vi "DriveReadEncoder.vi"(8 "error in":errorcluster, 11 "ModualNamePrefix":i32) -> (0 "error out":errorcluster, 2 "SWERVE_DRIVE_MODULE_POSITION":T1={"Distance"=0.0, "Angle"={"VALUE"=0.0, "COS"=1.0, "SIN"=0.0}, "P"=FALSE} {"Angle"."SIN" format="%13.4f"; "Angle"."COS" format="%13.4f"; "Angle"."VALUE" format="%13.4f"}, 3 "SWERVE_DRIVE_MODULE_STATE":T3={"Speed"=0.0, "Angle"={"VALUE"=0.0, "COS"=1.0, "SIN"=0.0}} {"Angle"."SIN" format="%13.4f"; "Angle"."COS" format="%13.4f"; "Angle"."VALUE" format="%13.4f"})   [LabVIEW 2023]
uses:
  <vilib>/Rock Robotics/WPI/ThirdParty/JAS_Junk/TrajLib/TypeDef/SWERVE_DRIVE_MODULE_STATE.ctl
  <vilib>/Rock Robotics/WPI/ThirdParty/JAS_Junk/TrajLib/TypeDef/ROTATION2D.ctl
  <vilib>/Rock Robotics/WPI/ThirdParty/JAS_Junk/TrajLib/TypeDef/SWERVE_DRIVE_MODULE_POSITION.ctl
  <vilib>/Rock Robotics/WPI/ThirdParty/JAS_Junk/TrajLib/Conv_Deg_Radians.vi
  <vilib>/Rock Robotics/WPI/ThirdParty/JAS_Junk/TrajLib/Rotation2d_CreateAngle.vi
  DriveGlobal.vi
  <vilib>/Rock Robotics/WPI/ThirdParty/Phoenix-LabVIEW/CANCoder/CTRE_Phoenix_CANcoder_RefNumRegistryGet.vi
  <vilib>/Rock Robotics/WPI/MotorControl/WPI_MotorControlRefNum Registry Get.vi
  <vilib>/Rock Robotics/WPI/ThirdParty/JAS_Junk/TrajLib/Trajectory_Library.lvlib
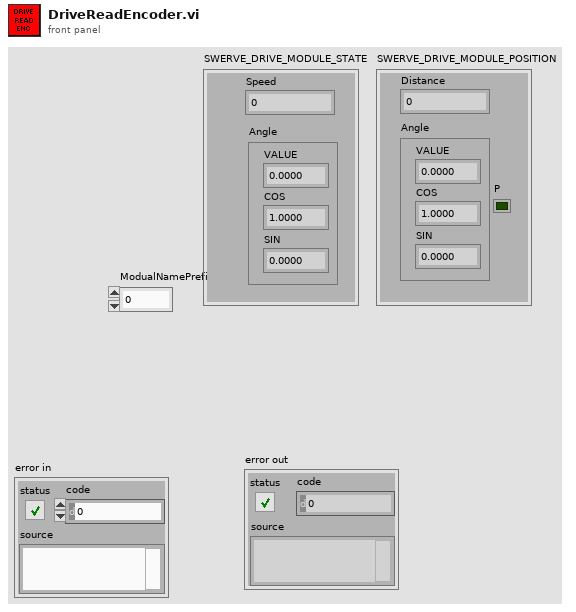
[diagram p1: front panel]
types:
  T1 = typedef "Trajectory_Library.lvlib/SWERVE_DRIVE_MODULE_POSITION.ctl" = cluster{"Distance":dbl, "Angle":T2, "P":bool}
  T2 = typedef "Trajectory_Library.lvlib/ROTATION2D.ctl" = cluster{"VALUE":dbl, "COS":dbl, "SIN":dbl}
  T3 = typedef "Trajectory_Library.lvlib/SWERVE_DRIVE_MODULE_STATE.ctl" = cluster{"Speed":dbl, "Angle":T2}
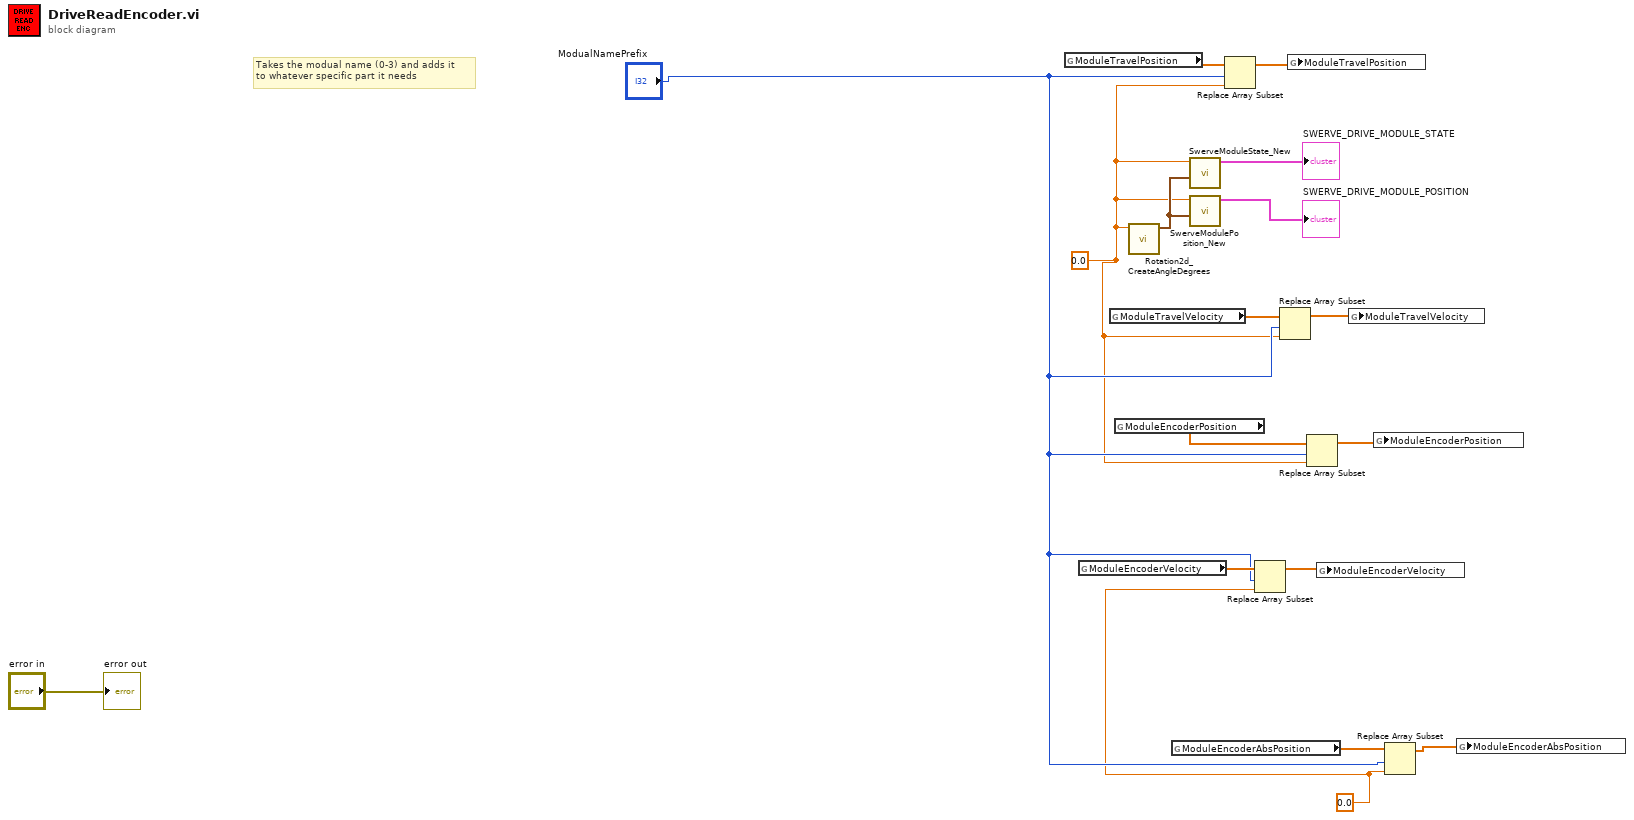
[diagram p0: block diagram]
diagram:
  w2 = 0.0 ("new element/subarray")
  w1 = 0.0 ("new element/subarray")
  # "Takes the modual name (0-3) and adds it \nto whatever specific part it needs"
  n1 = global read "DriveGlobal.vi" "ModuleTravelPosition"() -> (w13:dbl[])
  n2 = global read "DriveGlobal.vi" "ModuleEncoderVelocity"() -> (w7:dbl[])
  n3 = global read "DriveGlobal.vi" "ModuleTravelVelocity"() -> (w11:dbl[])
  n4 = global read "DriveGlobal.vi" "ModuleEncoderPosition"() -> (w9:dbl[])
  n5 = call <vilib>:"Rotation2d_CreateAngleDegrees.vi"("Angle_Degrees"=w2) -> ("ROTATION"=w16:T2)  [unwired: 10 in]
  n6 = global read "DriveGlobal.vi" "ModuleEncoderAbsPosition"() -> (w5:dbl[])
  n7 = call <vilib>:"SwerveModuleState_New.vi"("ROTATION"=w16, "Speed"=w2) -> ("SWERVE_DRIVE_MODULE_STATE"=→"SWERVE_DRIVE_MODULE_STATE":T3)  [unwired: 9 in]
  n8 = call <vilib>:"SwerveModulePosition_New.vi"("ROTATION"=w16, "Distance"=w2) -> ("SWERVE_DRIVE_MODULE_POSITION"=→"SWERVE_DRIVE_MODULE_POSITION":T1)  [unwired: 9 in]
  n9 = Replace Array Subset(array=w13, new element=w2, index="ModualNamePrefix") -> (w12:dbl[])
  n10 = Replace Array Subset(array=w7, new element=w1, index="ModualNamePrefix") -> (w6:dbl[])
  n11 = Replace Array Subset(array=w11, new element=w2, index="ModualNamePrefix") -> (w10:dbl[])
  n12 = global write "DriveGlobal.vi" "ModuleTravelPosition"(w12) -> ()
  n13 = Replace Array Subset(array=w9, new element=w2, index="ModualNamePrefix") -> (w8:dbl[])
  n14 = global write "DriveGlobal.vi" "ModuleEncoderVelocity"(w6) -> ()
  n15 = global write "DriveGlobal.vi" "ModuleTravelVelocity"(w10) -> ()
  n16 = global write "DriveGlobal.vi" "ModuleEncoderPosition"(w8) -> ()
  n17 = Replace Array Subset(array=w5, new element=w1, index="ModualNamePrefix") -> (w4:dbl[])
  n18 = global write "DriveGlobal.vi" "ModuleEncoderAbsPosition"(w4) -> ()
  "error out" <- "error in"
